vi "Reverse.vi"(11 "DAG in":refnum<class "DAG.lvclass">) -> (3 "reversed DAG":refnum<class "DAG.lvclass">)   [LabVIEW 2014, in "Raspberry Pi Compatible Compiler for LabVIEW.lvlib" / "DAG.lvclass"]
uses:
  DAG.lvclass
  DAG.lvclass/DAG.ctl
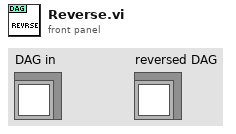
[diagram p1: front panel]
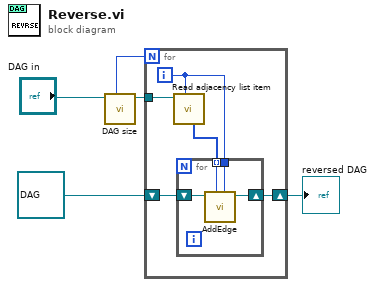
[diagram p0: block diagram]
diagram:
  n1 = call "DAG size.vi"("DAG in"="DAG in") -> ("DAG out"=w3:refnum<class "DAG.lvclass">, "vertices"=w4:i32)  [unwired: 6 in, 1 out]
  n2 = for {
    N: w4 -> [_]
    tunnel: w3 -> [w9]
    shift-right: [w7] -> w1
    shift-left: refnum<class "DAG.lvclass"> refnum ("reversed DAG") -> [w10]
    i -> [w8]
    n3 = call "Read adjacency list item.vi"("vertex"=w8, "DAG in"=w9) -> ("edge list"=w6:i32[])  [unwired: 6 in, 1 out]
    n4 = for {
      tunnel: w8 -> [w13]
      shift-right: [w12] -> w7
      shift-left: w10 -> [w14]
      tunnel: w6 -> [w11] mode=indexing
      n5 = call "AddEdge.vi"("end"=w13, "start"=w11, "DAG in"=w14) -> ("DAG out"=w12:refnum<class "DAG.lvclass">)  [unwired: 6 in]
    }
  }
  "reversed DAG" <- w1
